vi "Add AI Register.vi"(8 "error in (no error)":errorcluster, 9 "Mapping":T1={"DataType"=enum."U16", "Starting Address"=0, "Sub-Index (Bool)"=0, "VS Reference"=0}, 10 "Label":string="Input Register", 11 "Node Ref In":T3 format="%.0x") -> (0 "error out":errorcluster, 2 "Channel Ref out":T3 format="%.0x", 3 "Node Ref out":T3 format="%.0x")   [LabVIEW 2020, in "Modbus Master System Explorer.lvlib"]
uses:
  Modbus Master System Explorer.lvlib
  <vilib>/NI VeriStand/Custom Device API/Custom Device Item Ref.ctl
  Shared/Controls/Data Model/Mapping.ctl
  Shared/Controls/Data Model/DataType.ctl
  <vilib>/NI VeriStand/Custom Device API/Custom Device Channel.ctl
  <vilib>/NI VeriStand/Custom Device API/Custom Device Channel Type.ctl
  Modbus Type.ctl
  Radix.ctl
  Shared/Constants.vi
  <vilib>/NI VeriStand/Custom Device API/Custom Device API.lvlib
  Shared/Modbus Master Shared.lvlib
  <vilib>/NI VeriStand/Custom Device Tools/Custom Device Utility Library/Custom Device Utility Library.lvlib
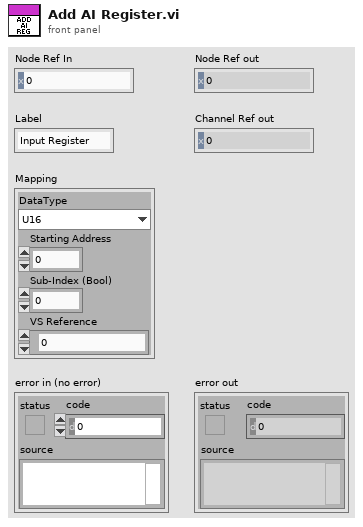
[diagram p1: front panel]
types:
  T1 = typedef "Modbus Master Shared.lvlib/Mapping.ctl" = cluster{"DataType":T2, "Starting Address":u16, "Sub-Index (Bool)":u16, "VS Reference":T3}
  T2 = typedef "Modbus Master Shared.lvlib/DataType.ctl" = enum16{"Double", "Single", "I64", "I32", "I16", "I8", "U64", "U32", "U16", "U8", "Boolean"}
  T3 = typedef "Custom Device API.lvlib/Custom Device Item Ref.ctl" = u64
  T4 = typedef "Modbus Master System Explorer.lvlib/Radix.ctl" = enum32{"Decimal", "Hexidecimal"}
  T5 = typedef "Custom Device API.lvlib/Custom Device Channel Type.ctl" = enum16{"Input", "Output"}
  T6 = typedef "Modbus Master Shared.lvlib/Modbus Type.ctl" = enum16{"Coil", "Discrete Input", "Holding Register", "Input Register"}
  T7 = typedef "Custom Device API.lvlib/Custom Device Channel.ctl" = cluster{"Type":T5, "Units":string, "Default Value":dbl, "Faultable":bool, "Scalable":bool}
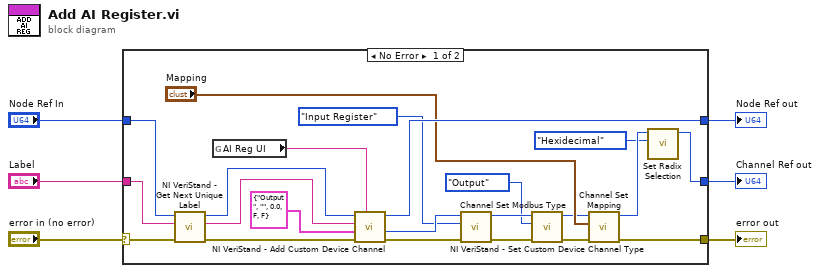
[diagram p0: block diagram]
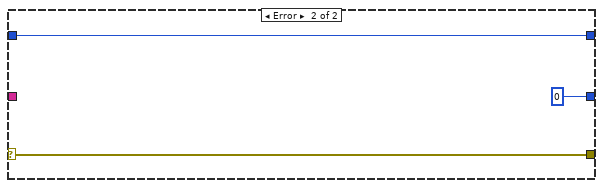
[diagram p2: hidden frame]
diagram:
  n1 = case shown="No Error" "error in (no error)" {
    selector: "error in (no error)" -> [w22 w30]
    tunnel: "Node Ref In" -> [w24 w31]
    tunnel: [w20 w31] -> w4
    tunnel: [w19 w30] -> w3
    tunnel: [w8 T3 0 ("Item Ref out")] -> w2
    tunnel: "Label" -> [w21 _]
    frame No Error {
      n2 = call <vilib>:"NI VeriStand - Get Next Unique Label.vi"("error in (no error)"=w22, "Label"=w21, "Parent Ref in"=w24) -> ("error out"=w26:errorcluster, "Label out"=w27:string, "Parent Ref dup"=w25:T3)  [unwired: 5 in, 1 out]
      n3 = global read "Constants.vi" "AI Reg UI"() -> (w23:string)
      n4 = call <vilib>:"NI VeriStand - Add Custom Device Channel.vi"("GUID (Default Channel)"=w23, "error in (no error)"=w26, "Channel"=T7 {"Type"=enum."Output", "Units"="", "Default Value"=0.0, "Faultable"=FALSE, "Scalable"=FALSE}, "Channel Name"=w27, "Parent Ref in"=w25) -> ("error out"=w17:errorcluster, "Channel Ref"=w16:T3, "Parent Ref out"=w20:T3)  [unwired: 3 in, 1 out]
      n5 = call "Channel Set Modbus Type.vi"("error in (no error)"=w17, "Type"=Modbus_Type."Input Register", "Channel Ref"=w16) -> ("error out"=w14:errorcluster, "Item Ref out"=w12:T3)  [unwired: 7 in]
      n6 = call <vilib>:"NI VeriStand - Set Custom Device Channel Type.vi"("error in (no error)"=w14, "Type"=Custom_Device_Channel_Type."Output", "Channel Ref in"=w12) -> ("error out"=w13:errorcluster, "Channel Ref out"=w11:T3)  [unwired: 7 in]
      n7 = call "Channel Set Mapping.vi"("error in (no error)"=w13, "Mapping"="Mapping", "Item Ref in"=w11) -> ("error out"=w19:errorcluster, "Item Ref out"=w9:T3)  [unwired: 7 in]
      n8 = call "Set Radix Selection.vi"("Radix"=Radix."Hexidecimal", "Item Ref in"=w9) -> ("Item Ref out"=w8:T3)  [unwired: 8 in, 1 out]
    }
    frame Error {
    }
  }
  "error out" <- w3
  "Node Ref out" <- w4
  "Channel Ref out" <- w2
